vi "Get Switch State.vi"(0 "VISA resource name":refnum<visa-resource-name>, 11 "error in (no error)":errorcluster) -> (4 "VISA resource name out":refnum<visa-resource-name>, 8 "Switch State":string, 15 "error out":errorcluster)   [LabVIEW 2023, in "ACM Visa Driver.lvlib"]
uses:
  ACM Visa Driver.lvlib
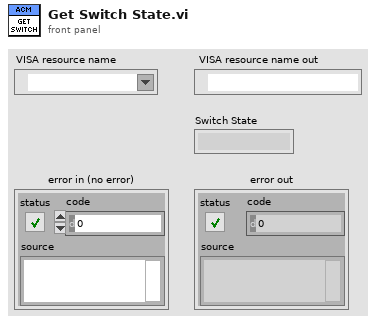
[diagram p1: front panel]
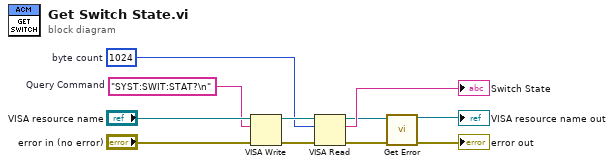
[diagram p0: block diagram]
diagram:
  w5 = u32 1024  # byte count
  w8 = "SYST:SWIT:STAT?\n"  # Query Command
  n1 = VISA Write(VISA resource name="VISA resource name", write buffer=w8, error in (no error)="error in (no error)") -> (VISA resource name out=w6:refnum<visa-resource-name>, error out=w10:errorcluster)  [unwired: 1 out]
  n2 = VISA Read(VISA resource name=w6, byte count=w5, error in (no error)=w10) -> (VISA resource name out=w2:refnum<visa-resource-name>, read buffer=→"Switch State":string, error out=w7:errorcluster)  [unwired: 1 out]
  n3 = call "Get Error.vi"("VISA resource name"=w2, "error in (no error)"=w7) -> ("VISA resource name out"=→"VISA resource name out":refnum<visa-resource-name>, "error out"=→"error out":errorcluster)  [unwired: 12 in]
